vi "ParseString.vi"(8 "error in (no error)":errorcluster, 10 "Index In":i32, 11 "JSON String":string) -> (0 "error out":errorcluster, 1 "Parsed String":string, 2 "Index Out":i32, 3 "JSON Tree":variant)   [LabVIEW 2013, in "i3-json.lvlib"]
doc: "Use this template to build a VI to use as a subVI."
uses:
  i3-json.lvlib
  JSON Types/JSON Type.ctl
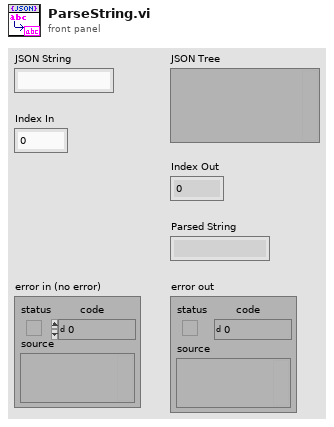
[diagram p1: front panel]
types:
  T1 = typedef "i3-json.lvlib/JSON Type.ctl" = enum8{"JSON Compatible", "JSON Array", "JSON Object", "JSON Null", "Double", "String", "Boolean", "Unknown"}
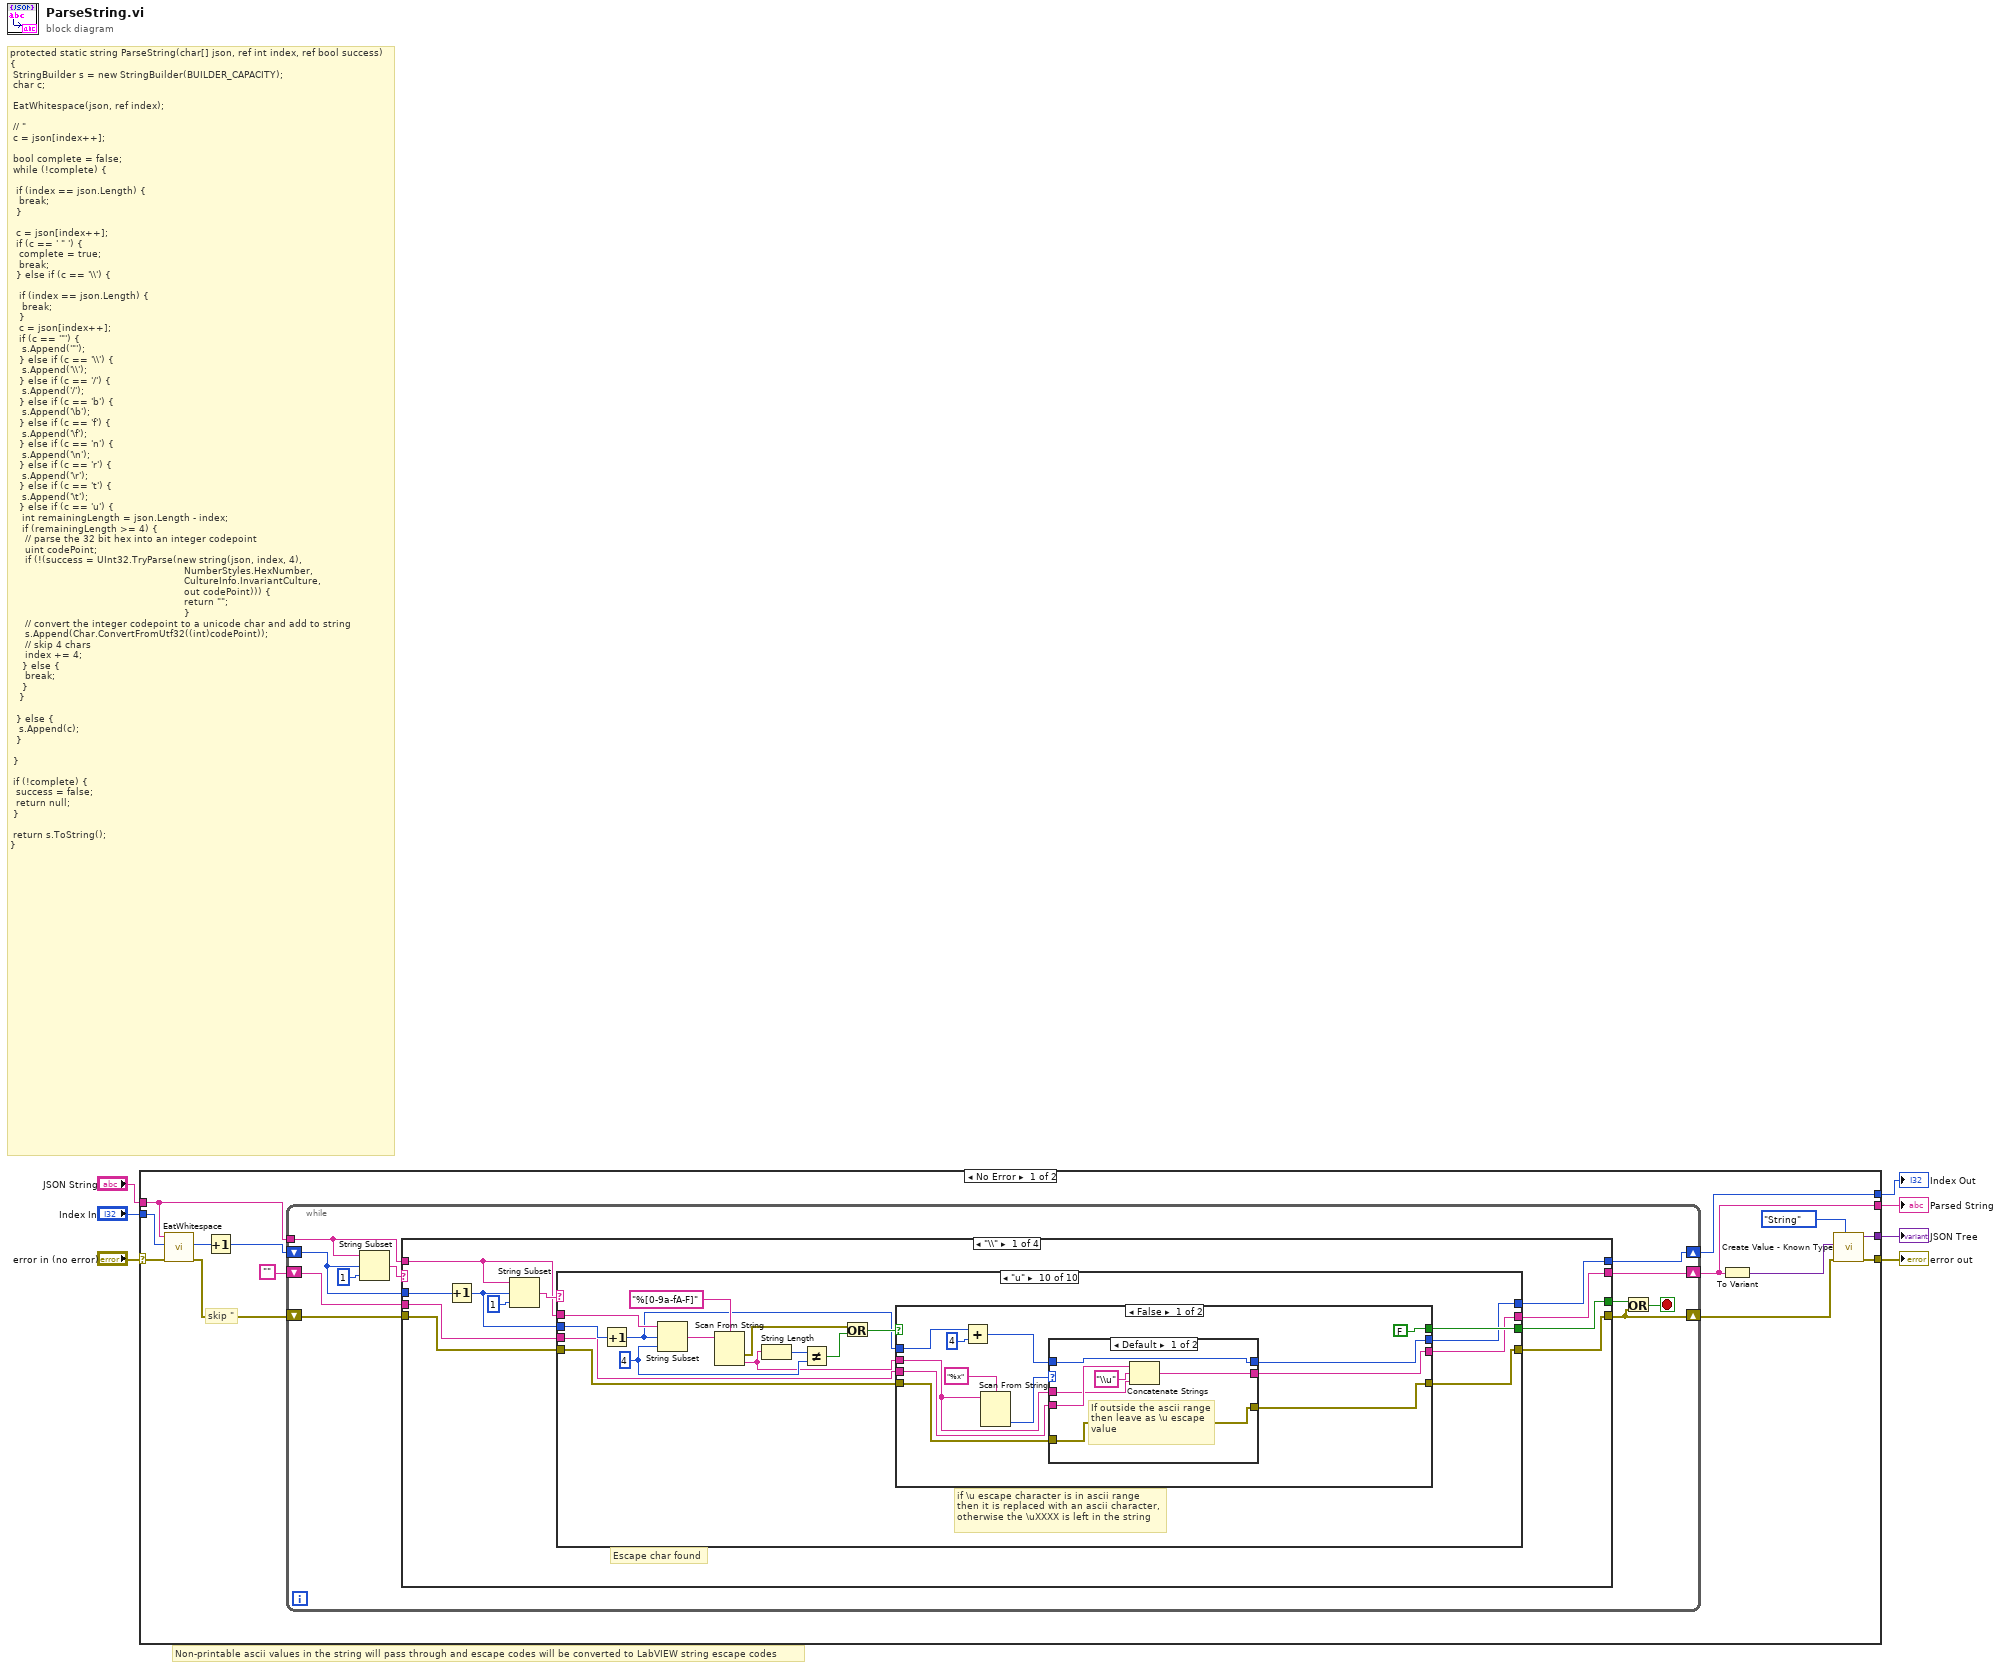
[diagram p0: block diagram]
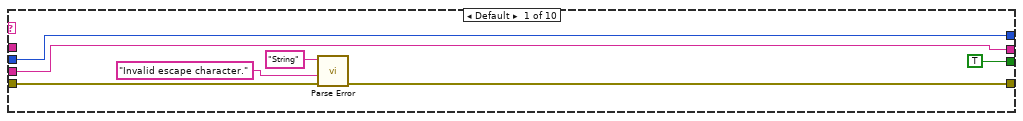
[diagram p2: hidden frame]
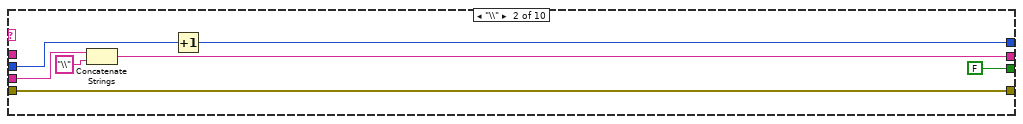
[diagram p3: hidden frame]
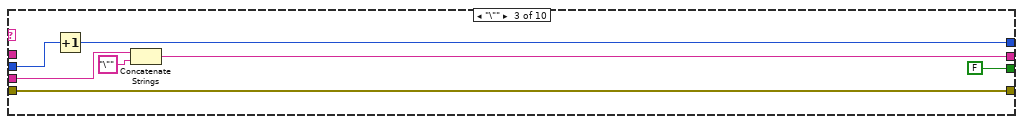
[diagram p4: hidden frame]
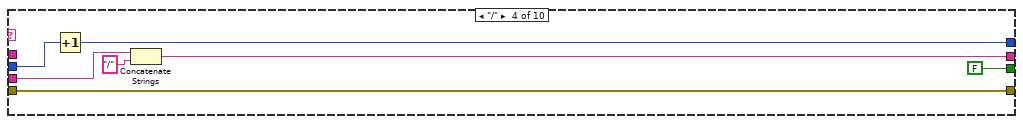
[diagram p5: hidden frame]
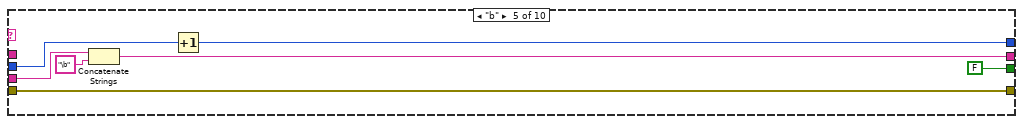
[diagram p6: hidden frame]
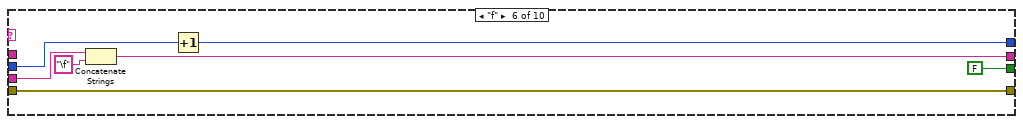
[diagram p7: hidden frame]
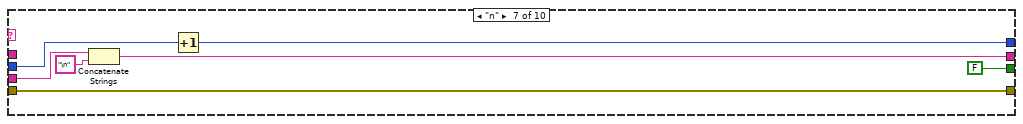
[diagram p8: hidden frame]
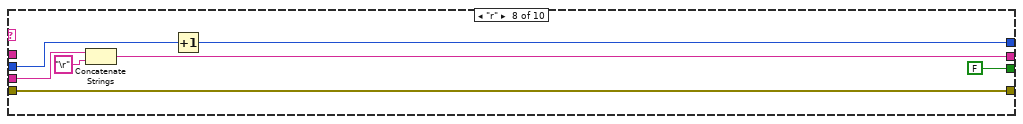
[diagram p9: hidden frame]
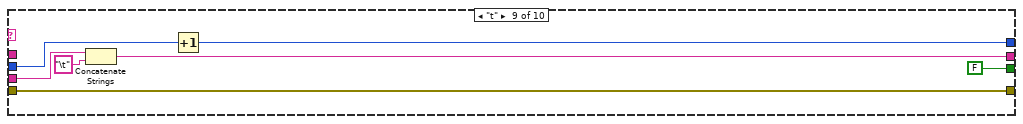
[diagram p10: hidden frame]
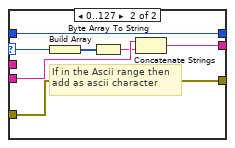
[diagram p11: hidden frame]
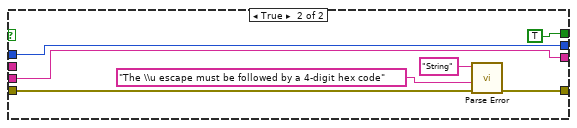
[diagram p12: hidden frame]
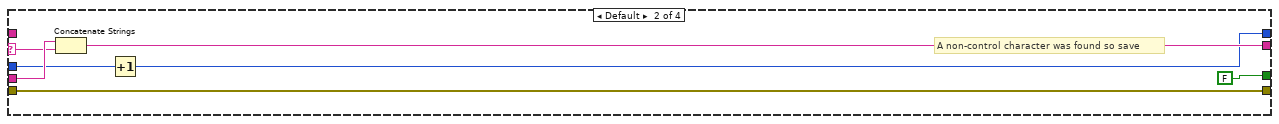
[diagram p13: hidden frame]
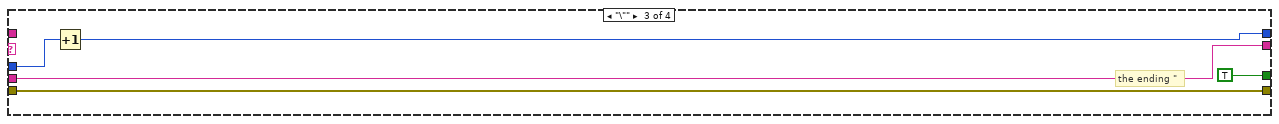
[diagram p14: hidden frame]
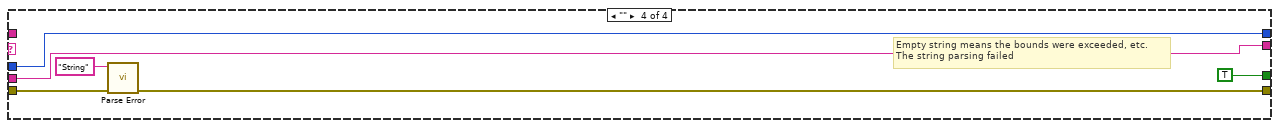
[diagram p15: hidden frame]
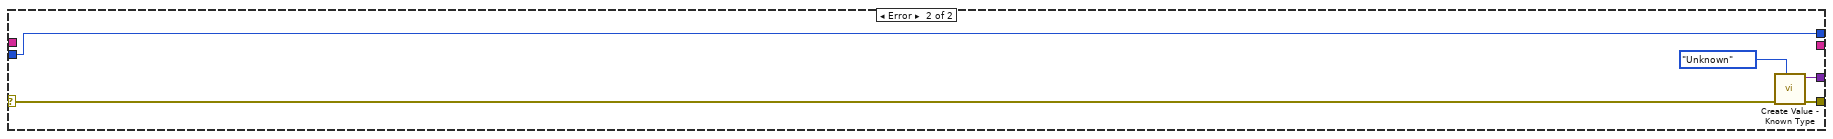
[diagram p16: hidden frame]
diagram:
  # "Non-printable ascii values in the string will pass through and escape codes will be converted to LabVIEW string escape codes"
  # "protected static string ParseString(char[] json, ref int index, ref bool success)\n{\n\tStringBuilder s = new StringBuilder(BUILDER_CAPACITY);\n\tchar c;\n\n\tEatWhitespace(json, ref index);\n\n\t// \"\n\tc = json[index++];\n\n\tbool complete = false;\n\twhile (!complete) {\n\n\t\tif (index == json.Length) {\n\t\t\tbreak;\n\t\t}\n\n\t\tc = json[index++];\n\t\tif (c == ' \" ') {\n\t\t\tcomplete = true;\n\t\t\tbreak;\n\t\t} else if (c == '\\\\') {\n\n\t\t\tif (index == json.Length) {\n\t\t\t\tbreak;\n\t\t\t}\n\t\t\tc = json[index++];\n\t\t\tif (c == '\"') {\n\t\t\t\ts.Append('\"');\n\t\t\t} else if (c == '\\\\') {\n\t\t\t\ts.Append('\\\\');\n\t\t\t} else if (c == '/') {\n\t\t\t\ts.Append('/');\n\t\t\t} else if (c == 'b') {\n\t\t\t\ts.Append('\\b');\n\t\t\t} else if (c == 'f') {\n\t\t\t\ts.Append('\\f');\n\t\t\t} else if (c == 'n') {\n\t\t\t\ts.Append('\\n');\n\t\t\t} else if (c == 'r') {\n\t\t\t\ts.Append('\\r');\n\t\t\t} else if (c == 't') {\n\t\t\t\ts.Append('\\t');\n\t\t\t} else if (c == 'u') {\n\t\t\t\tint remainingLength = json.Length - index;\n\t\t\t\tif (remainingLength >= 4) {\n\t\t\t\t\t// parse the 32 bit hex into an integer codepoint\n\t\t\t\t\tuint codePoint;\n\t\t\t\t\tif (!(success = UInt32.TryParse(new string(json, index, 4),\n                                                          NumberStyles.HexNumber,\n                                                          CultureInfo.InvariantCulture,\n                                                          out codePoint))) {\n\t\t\t\t\t\t                                                    return \"\";\n\t\t\t\t\t                                                     }\n\t\t\t\t\t// convert the integer codepoint to a unicode char and add to string\n\t\t\t\t\ts.Append(Char.ConvertFromUtf32((int)codePoint));\n\t\t\t\t\t// skip 4 chars\n\t\t\t\t\tindex += 4;\n\t\t\t\t} else {\n\t\t\t\t\tbreak;\n\t\t\t\t}\n\t\t\t}\n\n\t\t} else {\n\t\t\ts.Append(c);\n\t\t}\n\n\t}\n\n\tif (!complete) {\n\t\tsuccess = false;\n\t\treturn null;\n\t}\n\n\treturn s.ToString();\n}"
  n1 = case shown="No Error" "error in (no error)" {
    selector: "error in (no error)" -> [w21 w174]
    tunnel: [w13 w175] -> w6
    tunnel: "Index In" -> [w16 w178]
    tunnel: [w15 w178] -> w4
    tunnel: [w11 w176] -> w3
    tunnel: [w9 _] -> w2
    tunnel: "JSON String" -> [w8 _]
    frame No Error {
      # "skip \""
      n2 = call "EatWhitespace.vi"("error in (no error)"=w21, "Index In"=w16, "JSON String"=w8) -> ("error out"=w17:errorcluster, "Index Out"=w20:i32)  [unwired: 6 in, 1 out]
      n3 = Increment(x=w20) -> (x+1=w19:i32)
      n4 = while {
        tunnel: w8 -> [w28]
        shift-right: [w29] -> w9
        shift-left: "" -> [w30]
        shift-right: [w25] -> w15
        shift-left: w19 -> [w26]
        shift-right: [w24] -> w14
        shift-left: w17 -> [w27]
        stop <- w22 stop-if-true
        n5 = String Subset(string=w28, offset (0)=w26, length (rest)=1 ("length (rest)")) -> (substring=w31:string)
        n6 = case shown="\"\\\\\"" w31 {
          selector: w31 -> [_ w161 _ _]
          tunnel: [w34 FALSE TRUE TRUE] -> w23
          tunnel: w30 -> [w40 w162 w166 w173]
          tunnel: [w39 w160 w166 w173] -> w29
          tunnel: w26 -> [w43 w159 w165 w171]
          tunnel: w28 -> [w33 _ _ _]
          tunnel: [w38 w158 w164 w171] -> w25
          tunnel: w27 -> [w36 w156 w163 w169]
          tunnel: [w35 w156 w163 w168] -> w24
          frame "\\" {
            # "Escape char found"
            n7 = Increment(x=w43) -> (x+1=w37:i32)
            n8 = String Subset(string=w33, offset (0)=w37, length (rest)=1 ("length (rest)")) -> (substring=w41:string)
            n9 = case shown="\"u\"" w41 {
              tunnel: w40 -> [w49 w57 w64 w71 w78 w85 w92 w99 w106 w114]
              tunnel: [w49 w56 w63 w70 w77 w84 w91 w98 w105 w110] -> w39
              tunnel: [w48 w53 w60 w67 w74 w81 w88 w95 w102 w108] -> w38
              tunnel: w37 -> [w48 w54 w61 w68 w75 w82 w89 w96 w103 w122]
              tunnel: w36 -> [w45 w52 w59 w66 w73 w80 w87 w94 w101 w113]
              tunnel: [w44 w52 w59 w66 w73 w80 w87 w94 w101 w112] -> w35
              tunnel: [TRUE FALSE FALSE FALSE FALSE FALSE FALSE FALSE FALSE w111] -> w34
              tunnel: w33 -> [_ _ _ _ _ _ _ _ _ w123]
              frame Default {
                n10 = call "Parse Error.vi"("error in (no error)"=w45, "additional info"="Invalid escape character.", "datatype"="String") -> ("error out"=w44:errorcluster)  [unwired: 8 in]
              }
              frame "\\" {
                n11 = Concatenate Strings(w57, "\\" ("string")) -> (w56:string)
                n12 = Increment(x=w54) -> (x+1=w53:i32)
              }
              frame "\"" {
                n13 = Increment(x=w61) -> (x+1=w60:i32)
                n14 = Concatenate Strings(w64, "\"" ("string")) -> (w63:string)
              }
              frame "/" {
                n15 = Increment(x=w68) -> (x+1=w67:i32)
                n16 = Concatenate Strings(w71, "/" ("string")) -> (w70:string)
              }
              frame "b" {
                n17 = Concatenate Strings(w78, "\b" ("string")) -> (w77:string)
                n18 = Increment(x=w75) -> (x+1=w74:i32)
              }
              frame "f" {
                n19 = Concatenate Strings(w85, "\f" ("string")) -> (w84:string)
                n20 = Increment(x=w82) -> (x+1=w81:i32)
              }
              frame "n" {
                n21 = Concatenate Strings(w92, "\n" ("string")) -> (w91:string)
                n22 = Increment(x=w89) -> (x+1=w88:i32)
              }
              frame "r" {
                n23 = Concatenate Strings(w99, "\r" ("string")) -> (w98:string)
                n24 = Increment(x=w96) -> (x+1=w95:i32)
              }
              frame "t" {
                n25 = Concatenate Strings(w106, "\t" ("string")) -> (w105:string)
                n26 = Increment(x=w103) -> (x+1=w102:i32)
              }
              frame "u" {
                w116 = 4 ("length (rest)")
                # "if \\u escape character is in ascii range\nthen it is replaced with an ascii character,\notherwise the \\uXXXX is left in the string"
                n27 = Increment(x=w122) -> (x+1=w109:i32)
                n28 = String Subset(string=w123, offset (0)=w109, length (rest)=w116) -> (substring=w121:string)
                n29 = Scan From String(format string="%[0-9a-fA-F]", input string=w121) -> (error out=w117:errorcluster, output 1=w107:string)  [unwired: 3 in, 2 out]
                n30 = String Length(string=w107) -> (length=w119:i32)
                n31 = Not Equal?(x=w119, y=w116) -> (x != y?=w118:bool)
                n32 = Or(x=w117, y=w118) -> (x .or. y?=w115:bool)
                n33 = case shown="False" w115 {
                  tunnel: w114 -> [w132 w154]
                  tunnel: w113 -> [w130 w151]
                  tunnel: [w129 w150] -> w112
                  tunnel: [FALSE TRUE] -> w111
                  tunnel: [w131 w154] -> w110
                  tunnel: w109 -> [w125 w153]
                  tunnel: [w128 w153] -> w108
                  tunnel: w107 -> [w127 _]
                  frame False {
                    n34 = Add(x=w125, y=4) -> (x+y=w124:i32)
                    n35 = Scan From String(format string="%x", input string=w127) -> (output 1=w133:u32)  [unwired: 3 in, 3 out]
                    n36 = case shown="Default" w133 {
                      selector: w133 -> [_ w148]
                      tunnel: w132 -> [w138 w146]
                      tunnel: [w139 w145] -> w131
                      tunnel: w130 -> [w140 w144]
                      tunnel: [w140 w144] -> w129
                      tunnel: [w141 w142] -> w128
                      tunnel: w127 -> [w136 _]
                      tunnel: w124 -> [w141 w142]
                      frame Default {
                        # "If outside the ascii range\nthen leave as \\u escape\nvalue"
                        n37 = Concatenate Strings(w138, "\\u" ("string"), w136) -> (w139:string)
                      }
                      frame 0..127 {
                        # "If in the Ascii range then\nadd as ascii character"
                        n38 = Build Array(w148) -> (w147:u32[])
                        n39 = Byte Array To String(unsigned byte array=w147) -> (string=w143:string)
                        n40 = Concatenate Strings(w146, w143) -> (w145:string)
                      }
                    }
                  }
                  frame True {
                    n41 = call "Parse Error.vi"("error in (no error)"=w151, "additional info"="The \\u escape must be followed by a 4-digit hex code" ("source"), "datatype"="String") -> ("error out"=w150:errorcluster)  [unwired: 8 in]
                  }
                }
              }
            }
          }
          frame Default {
            # "A non-control character was found so save"
            n42 = Concatenate Strings(w162, w161) -> (w160:string)
            n43 = Increment(x=w159) -> (x+1=w158:i32)
          }
          frame "\"" {
            # "the ending \""
            n44 = Increment(x=w165) -> (x+1=w164:i32)
          }
          frame "" {
            # "Empty string means the bounds were exceeded, etc.\nThe string parsing failed"
            n45 = call "Parse Error.vi"("error in (no error)"=w169, "datatype"="String") -> ("error out"=w168:errorcluster)  [unwired: 9 in]
          }
        }
        n46 = Or(x=w23, y=w24) -> (x .or. y?=w22:bool)
      }
      n47 = To Variant(anything=w9) -> (Variant=w12:variant)
      n48 = call "Create Value - Known Type.vi"("JSON Type"=JSON_Type."String", "error in (no error)"=w14, "Value"=w12) -> ("error out"=w13:errorcluster, "JSON Tree"=w11:variant)  [unwired: 7 in]
    }
    frame Error {
      n49 = call "Create Value - Known Type.vi"("JSON Type"=JSON_Type."Unknown", "error in (no error)"=w174) -> ("error out"=w175:errorcluster, "JSON Tree"=w176:variant)  [unwired: 8 in]
    }
  }
  "error out" <- w6
  "Index Out" <- w4
  "JSON Tree" <- w3
  "Parsed String" <- w2
